vi "GetProperty.vi"(7 "Property":string, 8 "error in":errorcluster, 11 "camera.nit in":refnum<class "camera.lvclass">) -> (0 "error out":errorcluster, 2 "value":string)   [LabVIEW 2020, in "camera.lvclass"]
uses:
  camera.lvclass
  camera.lvclass/camera.ctl
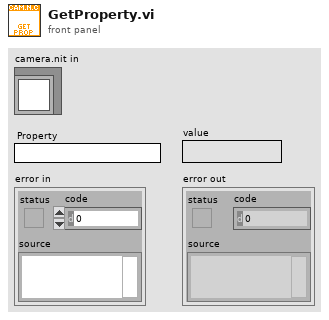
[diagram p1: front panel]
types:
  T1 = typedef "camera.lvclass/config.ctl" = cluster{"session":refnum<k35>, "path":path}
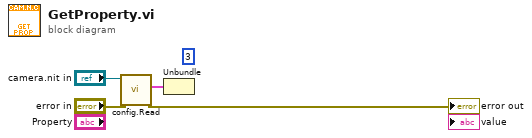
[diagram p0: block diagram]
diagram:
  (unwired) 3
  n1 = call "config.Read.vi"("error in"="error in", "camera.nit in"="camera.nit in") -> ("error out"=→"error out":errorcluster, "data value"=w3:T1)  [unwired: 8 in]
  n2 = Unbundle(w3) -> ()  [unwired: 2 out]
